vi "Extract Word.vi"(8 "error in (no error)":errorcluster, 11 "file path (use dialog)":path) -> (0 "error out":errorcluster, 3 "Random Word":string)   [LabVIEW 2018]
panel:
  out "Array Size":i32
  in  "Pick!":bool
  in  "Stop":bool
  out "Duplicates Removed":string[](array[string])
  out "Long words only":string[](array[string])
  out "Capitalized words removed":string[](array[string])
  out "punctuation removed":string
  out "Empty elements removed":string[](array[string])
  out "Separated by spaces":string[](array[string])
  out "Newlines removed":string
  out "Full Text":string
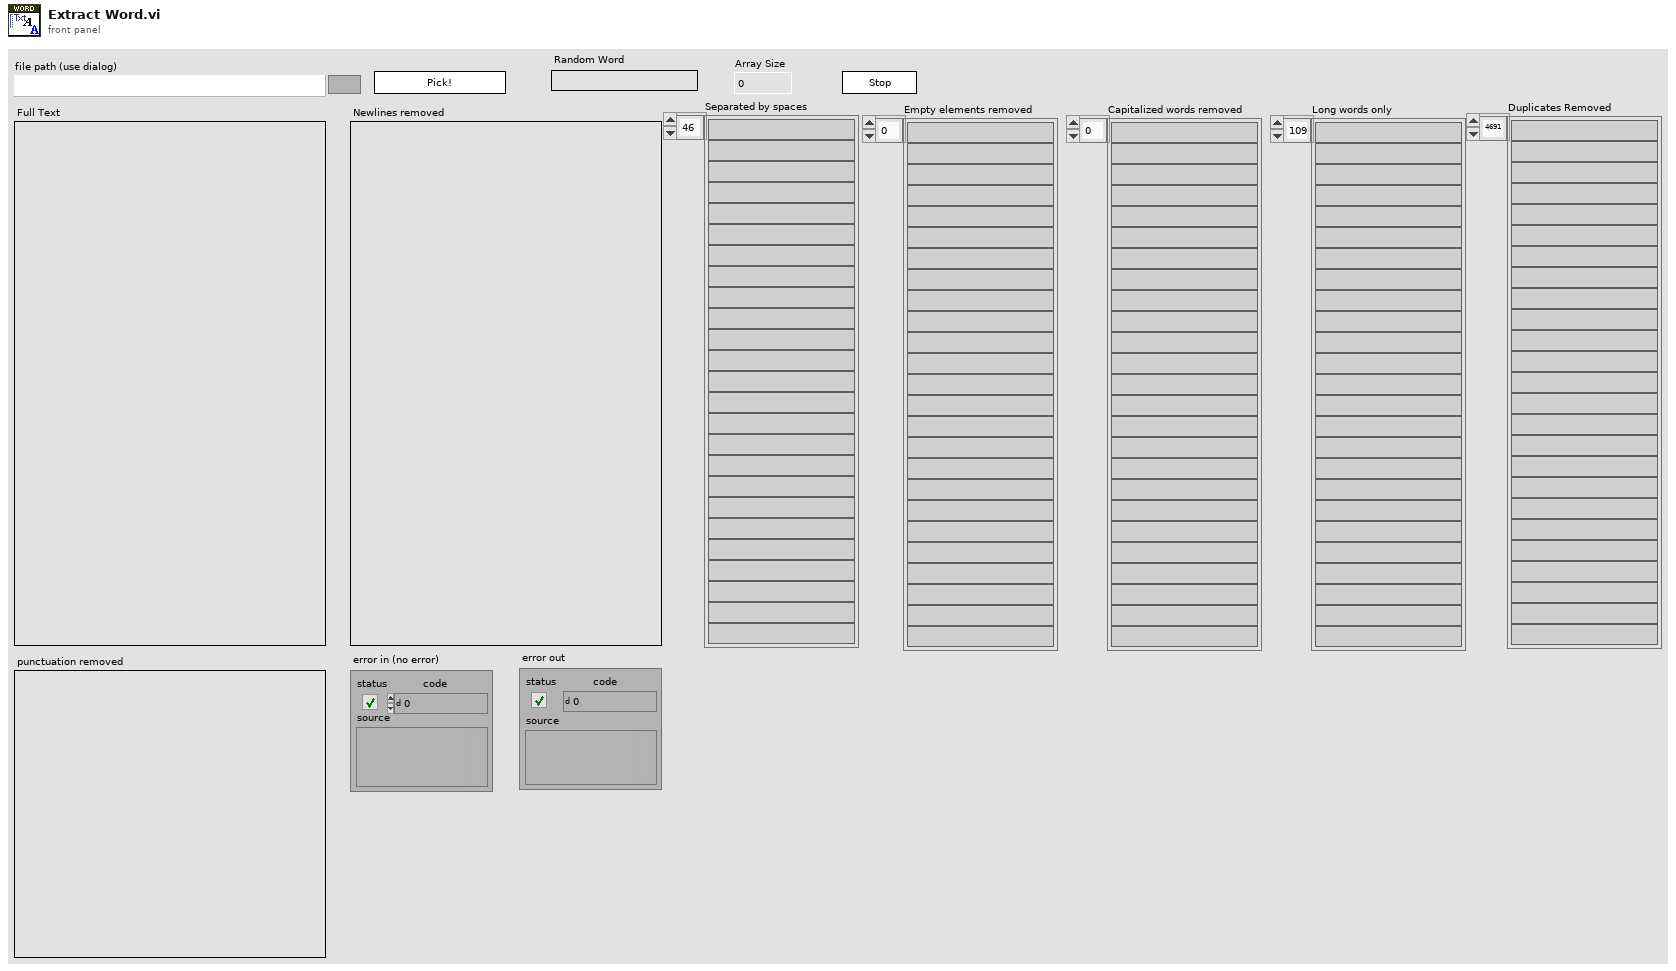
[diagram p1: front panel]
types:
  T1 = enum32{"Bad", "Idle", "Run top level", "Running"}
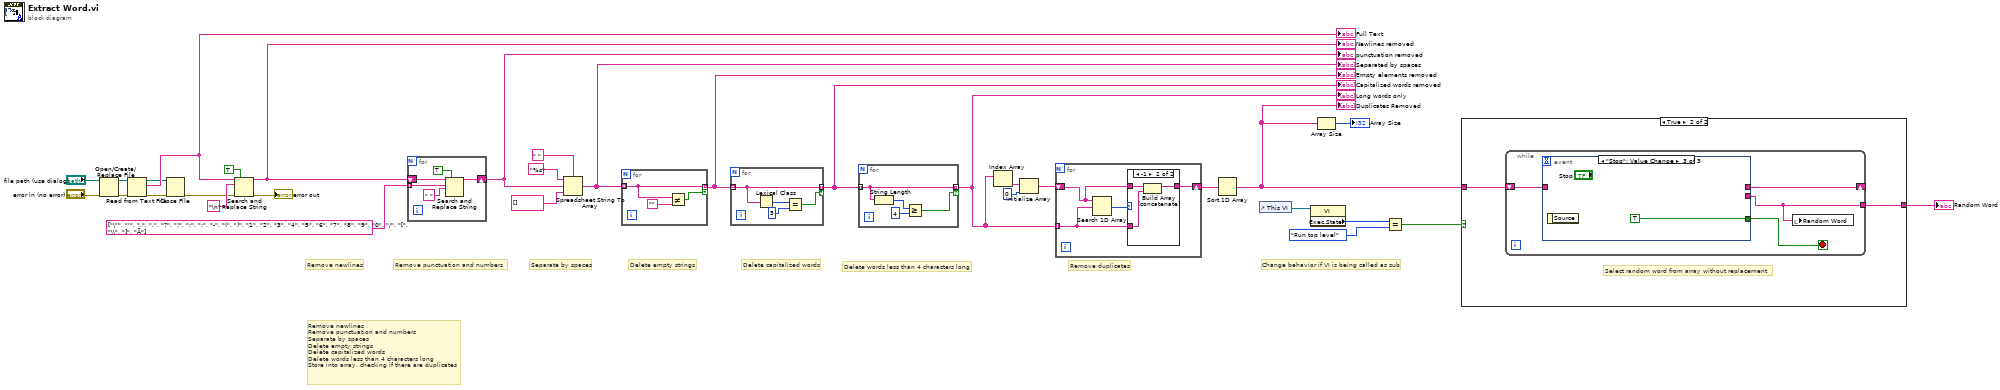
[diagram p0: block diagram]
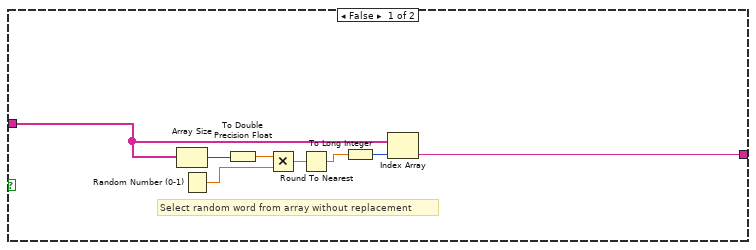
[diagram p2: hidden frame]
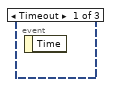
[diagram p3: hidden frame]
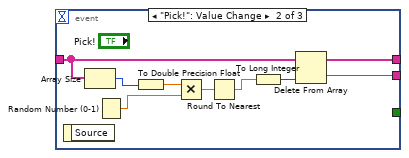
[diagram p4: hidden frame]
diagram:
  # "Change behavior if VI is being called as sub"
  # "Remove duplicates"
  # "Delete words less than 4 characters long"
  # "Delete capitalized words"
  # "Remove punctuation and numbers"
  # "Delete empty strings"
  # "Separate by spaces"
  # "Remove newlines"
  # "Remove newlines\nRemove punctuation and numbers\nSeparate by spaces\nDelete empty strings\nDelete capitalized words\nDelete words less than 4 characters long\nStore into array, checking if there are duplicates"
  n1 = Open/Create/Replace File(file path (use dialog)="file path (use dialog)", error in="error in (no error)") -> (refnum out=w31:refnum<file>, error out=w30:errorcluster)  [unwired: 4 in, 1 out]
  n2 = Read from Text File(file (use dialog)=w31, error in=w30) -> (refnum out=w1:refnum<file>, text=w29:string, error out=w27:errorcluster)  [unwired: 2 in, 1 out]
  "Full Text" <- w29
  n3 = Close File(refnum=w1, error in=w27) -> (error out=w2:errorcluster)  [unwired: 1 out]
  n4 = Search and Replace String(replace all?=TRUE ("replace all? (F)"), input string=w29, search string="\n", error in=w2) -> (result string=w22:string, error out=→"error out":errorcluster)  [unwired: 4 in, 2 out]
  "Newlines removed" <- w22
  n5 = for {
    tunnel: string[] ["\"", "'", ",", ".", "?", "!", ";", ":", "-", "(", ")", "1", "2", "3", "4", "5", "6", "7", "8", "9", "0", "/", "[", "\\", "]", "Ã"] -> [w35] mode=indexing
    shift-right: [w34] -> w20
    shift-left: w22 -> [w37]
    n6 = Search and Replace String(replace all?=TRUE ("replace all? (F)"), input string=w37, search string=w35, replace string=" " ("replace string (\"\")")) -> (result string=w34:string)  [unwired: 4 in, 3 out]
  }
  "punctuation removed" <- w20
  n7 = Spreadsheet String To Array(delimiter (Tab)=" ", format string="%s", spreadsheet string=w20, array type (2D Dbl)=string[] []) -> (array=w12:string[])
  "Separated by spaces" <- w12
  n8 = for {
    tunnel: w12 -> [w40] mode=indexing
    tunnel: [w40] -> w11 mode=indexing if=w39
    n9 = Not Equal?(x=w40, y="") -> (x != y?=w39:bool)
  }
  "Empty elements removed" <- w11
  n10 = for {
    tunnel: w11 -> [w42] mode=indexing
    tunnel: [w42] -> w19 mode=indexing if=w41
    n11 = Lexical Class(1:w42) -> (0:w44:i16)
    n12 = Equal?(x=w44, y=i16 5) -> (x = y?=w41:bool)
  }
  "Capitalized words removed" <- w19
  n13 = for {
    tunnel: w19 -> [w46] mode=indexing
    tunnel: [w46] -> w18 mode=indexing if=w45
    n14 = String Length(string=w46) -> (length=w48:i32)
    n15 = Greater Or Equal?(x=w48, y=4) -> (x >= y?=w45:bool)
  }
  "Long words only" <- w18
  n16 = Index Array(array=w18) -> (element=w17:string)  [unwired: 1 in]
  n17 = Initialize Array(w17, 0 ("dimension size")) -> (w16:string[])
  n18 = for {
    tunnel: w18 -> [w49] mode=indexing
    shift-right: [w51] -> w14
    shift-left: w16 -> [w52]
    n19 = Search 1D Array(1D array=w52, element=w49) -> (index of element=w50:i32)  [unwired: 1 in]
    n20 = case shown="-1" w50 {
      tunnel: w52 -> [w53 w56]
      tunnel: [w53 w55] -> w51
      tunnel: w49 -> [_ w54]
      frame Default {
      }
      frame -1 {
        n21 = Build Array (concatenate)(w56, w54) -> (w55:string[])
      }
    }
  }
  n22 = Sort 1D Array(array=w14) -> (sorted array=w10:string[])
  "Duplicates Removed" <- w10
  n23 = control-ref of="This VI"() -> (w9:refnum<vi>)
  n24 = property class="VI"(reference=w9) -> ("Exec.State"=w8:T1)  [unwired: 1 in, 2 out]
  n25 = Array Size(array=w10) -> (size(s)=→"Array Size":i32)
  n26 = Equal?(x=w8, y=T1."Run top level") -> (x = y?=w6:bool)
  n27 = case shown="True" w6 {
    tunnel: w10 -> [w59 w66]
    tunnel: [w58 w65] -> w5
    frame False {
      # "Select random word from array without replacement"
      n28 = Array Size(array=w59) -> (size(s)=w64:i32)
      n29 = Random Number (0-1)() -> (number: 0 to 1=w63:dbl)
      n30 = To Double Precision Float(number=w64) -> (double precision float=w60:dbl)
      n31 = Multiply(x=w60, y=w63) -> (x*y=w62:dbl)
      n32 = Round To Nearest(number=w62) -> (nearest integer value=w61:dbl)
      n33 = To Long Integer(number=w61) -> (32bit integer=w57:i32)
      n34 = Index Array(array=w59, index=w57) -> (element=w58:string)
    }
    frame True {
      # "Select random word from array without replacement"
      n35 = while {
        shift-right: [w68] -> _
        shift-left: w66 -> [w70]
        tunnel: [w67] -> w65
        stop <- w69 stop-if-true
        n36 = event shown="[2] \"Stop\": Value Change" {
          selector: _ -> [_ _ _]
          dyn-events: _ -> [_ _ _]
          timeout: _ -> [_ _ _]
          tunnel: w70 -> [_ w79 _]
          tunnel: [_ _ TRUE] -> w69
          tunnel: [_ w78 _] -> w68
          tunnel: [_ w77 _] -> w67
          event Timeout {
            n37 = event-data() -> ()  [unwired: 1 in, 1 out]
          }
          event "Pick!": Value Change {
            n38 = event-data() -> ()  [unwired: 1 in, 1 out]
            n39 = Array Size(array=w79) -> (size(s)=w76:i32)
            n40 = Random Number (0-1)() -> (number: 0 to 1=w75:dbl)
            n41 = To Double Precision Float(number=w76) -> (double precision float=w71:dbl)
            n42 = Multiply(x=w71, y=w75) -> (x*y=w74:dbl)
            n43 = Round To Nearest(number=w74) -> (nearest integer value=w73:dbl)
            n44 = To Long Integer(number=w73) -> (32bit integer=w72:i32)
            n45 = Delete From Array(array=w79, index=w72) -> (deleted portion=w77:string, array with subset deleted=w78:string[])  [unwired: 1 in]
          }
          event "Stop": Value Change {
            n46 = event-data() -> ()  [unwired: 1 in, 1 out]
          }
        }
        n47 = local write "Random Word"(w67) -> ()
      }
    }
  }
  "Random Word" <- w5
